vi "Datalogger Path Set Message Create.vi"(8 "error in (no error)":errorcluster, 10 "Path":path, 11 "Datalogger Path Set in":refnum<class "Datalogger Path Set Message.lvclass">) -> (0 "error out":errorcluster, 3 "Datalogger Path Set out":refnum<class "Datalogger Path Set Message.lvclass">)   [LabVIEW 2018, in "Datalogger Path Set Message.lvclass"]
uses:
  Datalogger Path Set Message.lvclass
  Datalogger Path Set Message.lvclass/Datalogger Path Set Message.ctl
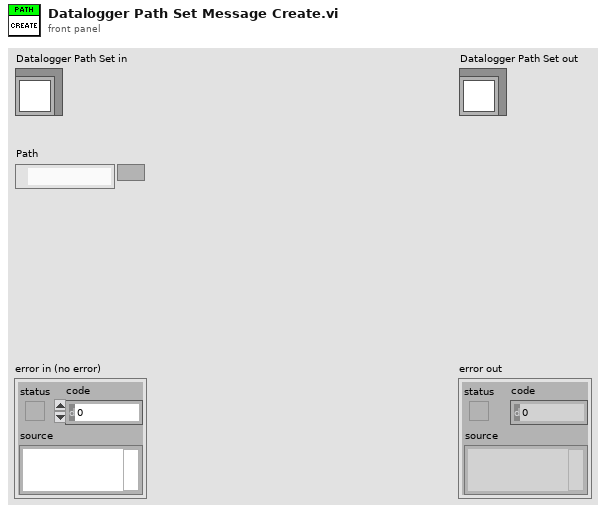
[diagram p1: front panel]
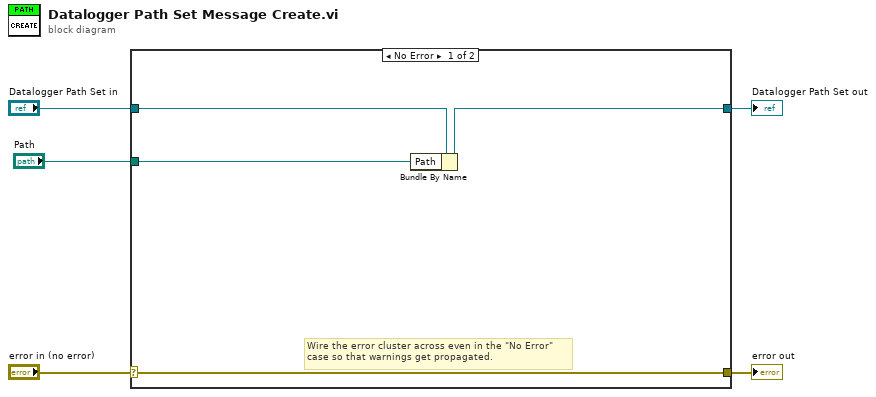
[diagram p0: block diagram]
diagram:
  n1 = case shown="No Error" "error in (no error)" {
    selector: "error in (no error)" -> [w9 w11]
    tunnel: [w9 w11] -> w4
    tunnel: [w6 w10] -> w2
    tunnel: "Datalogger Path Set in" -> [w8 w10]
    tunnel: "Path" -> [w7 _]
    frame No Error {
      # "Wire the error cluster across even in the \"No Error\"\ncase so that warnings get propagated."
      n2 = Bundle By Name(cluster=w8, "Path"=w7) -> (w6:refnum<class "Datalogger Path Set Message.lvclass">)
    }
    frame Error {
    }
  }
  "error out" <- w4
  "Datalogger Path Set out" <- w2
